vi "Asynchronous - Update Cyclic Labels Parameters Channels.vi"(5 "Channel Data []":T5[](array[typedef])=[{"Labels Settings"=[{"Name"="", "xmlName"="", "Label"=0, "transferPeriod"=0, "SDI_Enabled"=FALSE, "SDI"=0, "Word"={"Param Setting"={"Start Bit"=[], "Num Bits"=[], "Signed?"=[], "ScaleFac"=[], "ScaleOffset"=[], "Block Data Refs"=[], "Encoding"=[], "Values Array"=[], "Item Refs"=[]}}, "TransferType"=enum."ScheduledLabel", "has timestamp?"=FALSE, "Label Disable/Trigger Channel Reference"=0, "Message Handle"=0, "Initialized?"=FALSE, "Word Initial Raw Value"=0, "Label Timestamp Channel Data Reference"=0}], "channel handle"=0, "channel #"=0}] {"Labels Settings"."Label Timestamp Channel Data Reference" format="%.0x"; "Labels Settings"."Label Disable/Trigger Channel Reference" format="%.0x"; "Labels Settings"."Word"."Param Setting"."Item Refs" format="%.0x"; "Labels Settings"."Word"."Param Setting"."Num Bits" min=1 max=32; "Labels Settings"."Word"."Param Setting"."Start Bit" min=8 max=31; "Labels Settings"."Label" format="%.0o"}, 6 "core handle":u64, 7 "Map":T4[](array[typedef]) {"Channel Data Reference" format="%.0x"}, 8 "Error (in)":errorcluster, 9 "Updated FIFO Index []":i32[](array[numeric]), 10 "Doubles []":dbl[](array[numeric]), 11 "Raw Values":T1) -> (0 "Error (out)":errorcluster)   [LabVIEW 2020]
uses:
  Shared/Controls and Global/RT HW Channel.ctl
  Shared/Controls and Global/RT Label Settings.ctl
  Shared/Controls and Global/Label.ctl
  Shared/Controls and Global/transferPeriod.ctl
  Shared/Controls and Global/RT Word Settings.ctl
  Shared/Controls and Global/RT Param Setting.ctl
  Shared/Controls and Global/Start Bit.ctl
  Shared/Controls and Global/Number of Bits.ctl
  <vilib>/NI VeriStand/Custom Device API/Block Data Reference.ctl
  <vilib>/NI VeriStand/Custom Device API/Data Reference.ctl
  <vilib>/NI VeriStand/Custom Device API/Custom Device Item Ref.ctl
  Shared/Controls and Global/TransferType.ctl
  RT Controls/RT Tx Association.ctl
  RT Controls/RT Tx Default Raw Value.ctl
  RT Controls/RT Tx Default Raw Value_Association.ctl
  Insert BCD Parameter.vi
  Ballard Arinc-429 Engine.lvlib
  <instrlib>/BTI429Lib/BTI429LV.lvlib
  <vilib>/NI VeriStand/Custom Device Tools/Custom Device Utility Library/Custom Device Utility Library.lvlib
  Shared/Ballard Arinc-429 Shared.lvlib
  <vilib>/NI VeriStand/Custom Device API/Custom Device API.lvlib
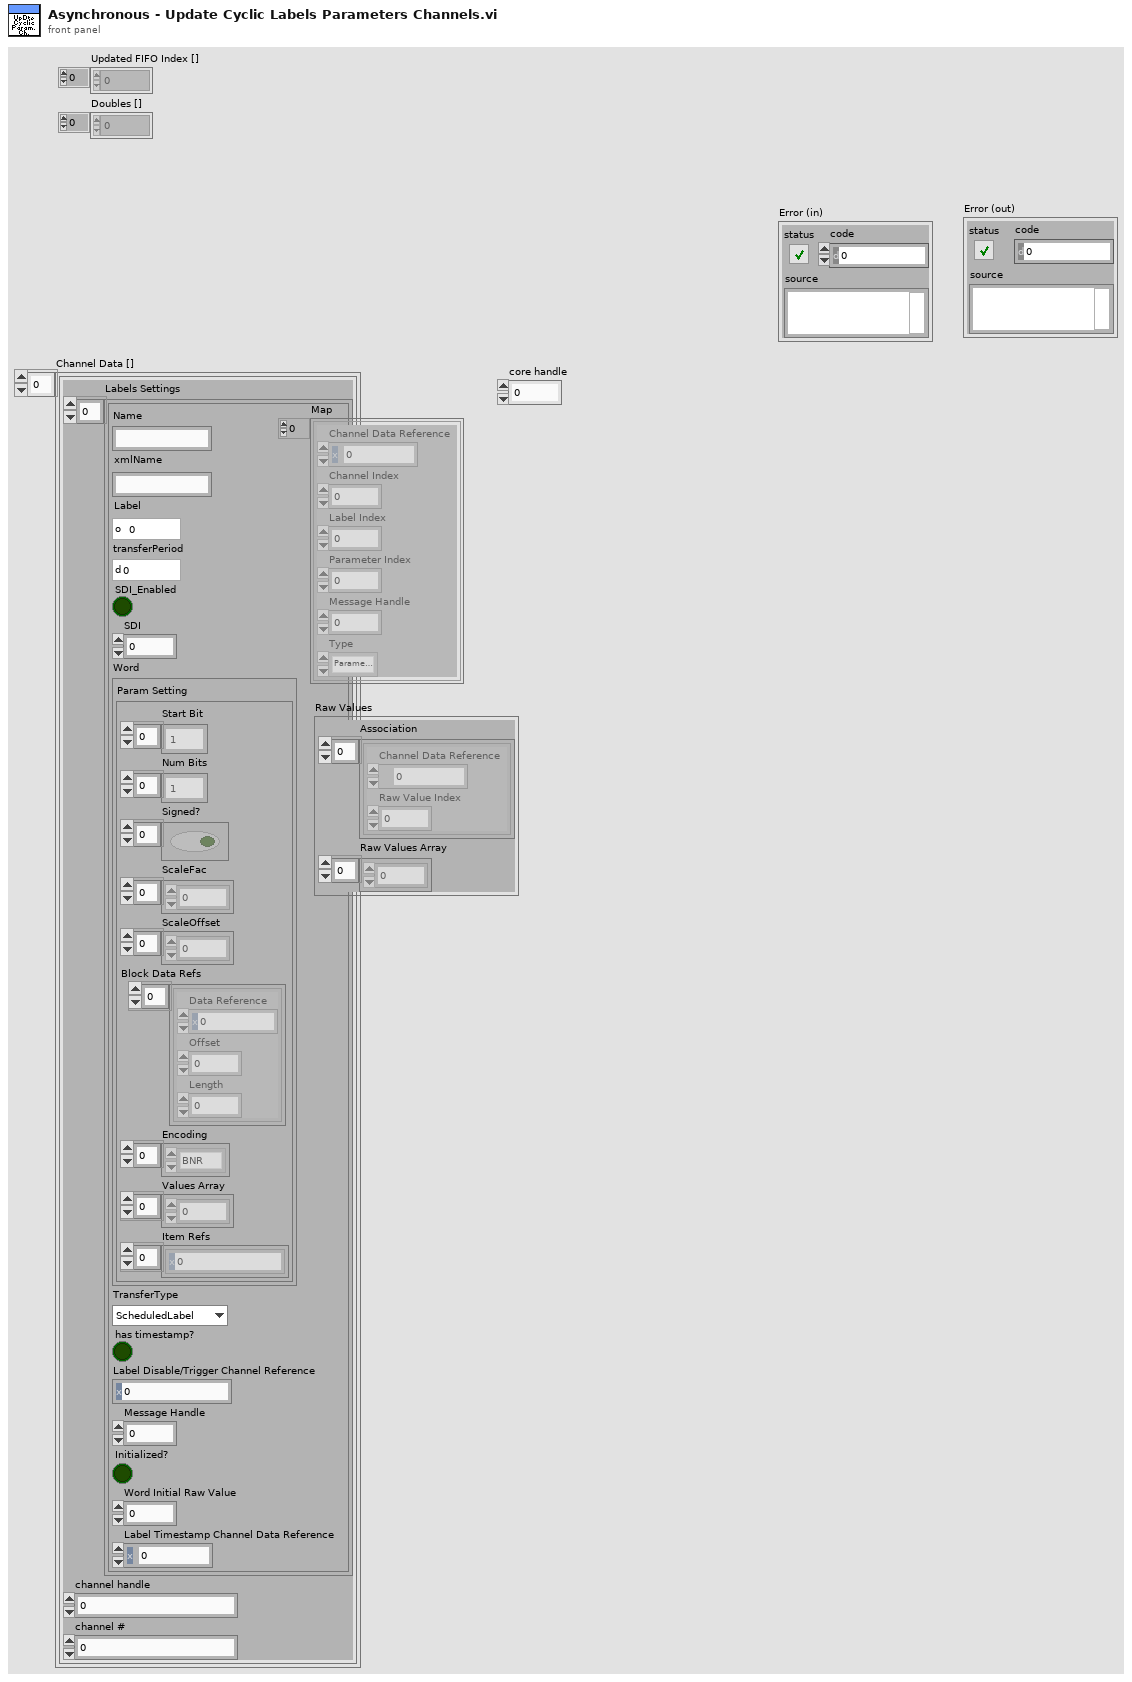
[diagram p1: front panel]
types:
  T1 = typedef "Ballard Arinc-429 Engine.lvlib/RT Tx Default Raw Value.ctl" = cluster{"Association":T2[], "Raw Values Array":u32[]}
  T2 = typedef "Ballard Arinc-429 Engine.lvlib/RT Tx Default Raw Value_Association.ctl" = cluster{"Channel Data Reference":T3, "Raw Value Index":i32}
  T3 = typedef "Custom Device API.lvlib/Data Reference.ctl" = i32
  T4 = typedef "Ballard Arinc-429 Engine.lvlib/RT Tx Association.ctl" = cluster{"Channel Data Reference":T3, "Channel Index":i32, "Label Index":i32, "Parameter Index":i32, "Message Handle":u64, "Type":enum16{"Parameter Channel", "Disable/Trigger Channel"}}
  T5 = typedef "Ballard Arinc-429 Shared.lvlib/RT HW Channel.ctl" = cluster{"Labels Settings":T6[], "channel handle":u64, "channel #":u16}
  T6 = typedef "Ballard Arinc-429 Shared.lvlib/RT Label Settings.ctl" = cluster{"Name":string, "xmlName":string, "Label":T7, "transferPeriod":T8, "SDI_Enabled":bool, "SDI":u8, "Word":T9, "TransferType":T15, "has timestamp?":bool, "Label Disable/Trigger Channel Reference":T14, "Message Handle":u64, "Initialized?":bool, "Word Initial Raw Value":u32, "Label Timestamp Channel Data Reference":T3}
  T7 = typedef "Ballard Arinc-429 Shared.lvlib/Label.ctl" = u8
  T8 = typedef "Ballard Arinc-429 Shared.lvlib/transferPeriod.ctl" = u32
  T9 = typedef "Ballard Arinc-429 Shared.lvlib/RT Word Settings.ctl" = cluster{"Param Setting":T10}
  T10 = typedef "Ballard Arinc-429 Shared.lvlib/RT Param Setting.ctl" = cluster{"Start Bit":T11[], "Num Bits":T12[], "Signed?":bool[], "ScaleFac":dbl[], "ScaleOffset":dbl[], "Block Data Refs":T13[], "Encoding":enum16{"BNR", "BCD", "Discrete"}[], "Values Array":dbl[], "Item Refs":T14[]}
  T11 = typedef "Ballard Arinc-429 Shared.lvlib/Start Bit.ctl" = i32
  T12 = typedef "Ballard Arinc-429 Shared.lvlib/Number of Bits.ctl" = i32
  T13 = typedef "Custom Device API.lvlib/Block Data Reference.ctl" = cluster{"Data Reference":T3, "Offset":u64, "Length":u64}
  T14 = typedef "Custom Device API.lvlib/Custom Device Item Ref.ctl" = u64
  T15 = typedef "Ballard Arinc-429 Shared.lvlib/TransferType.ctl" = enum16{"ScheduledLabel", "Acyclic", "Block", "Strobe"}
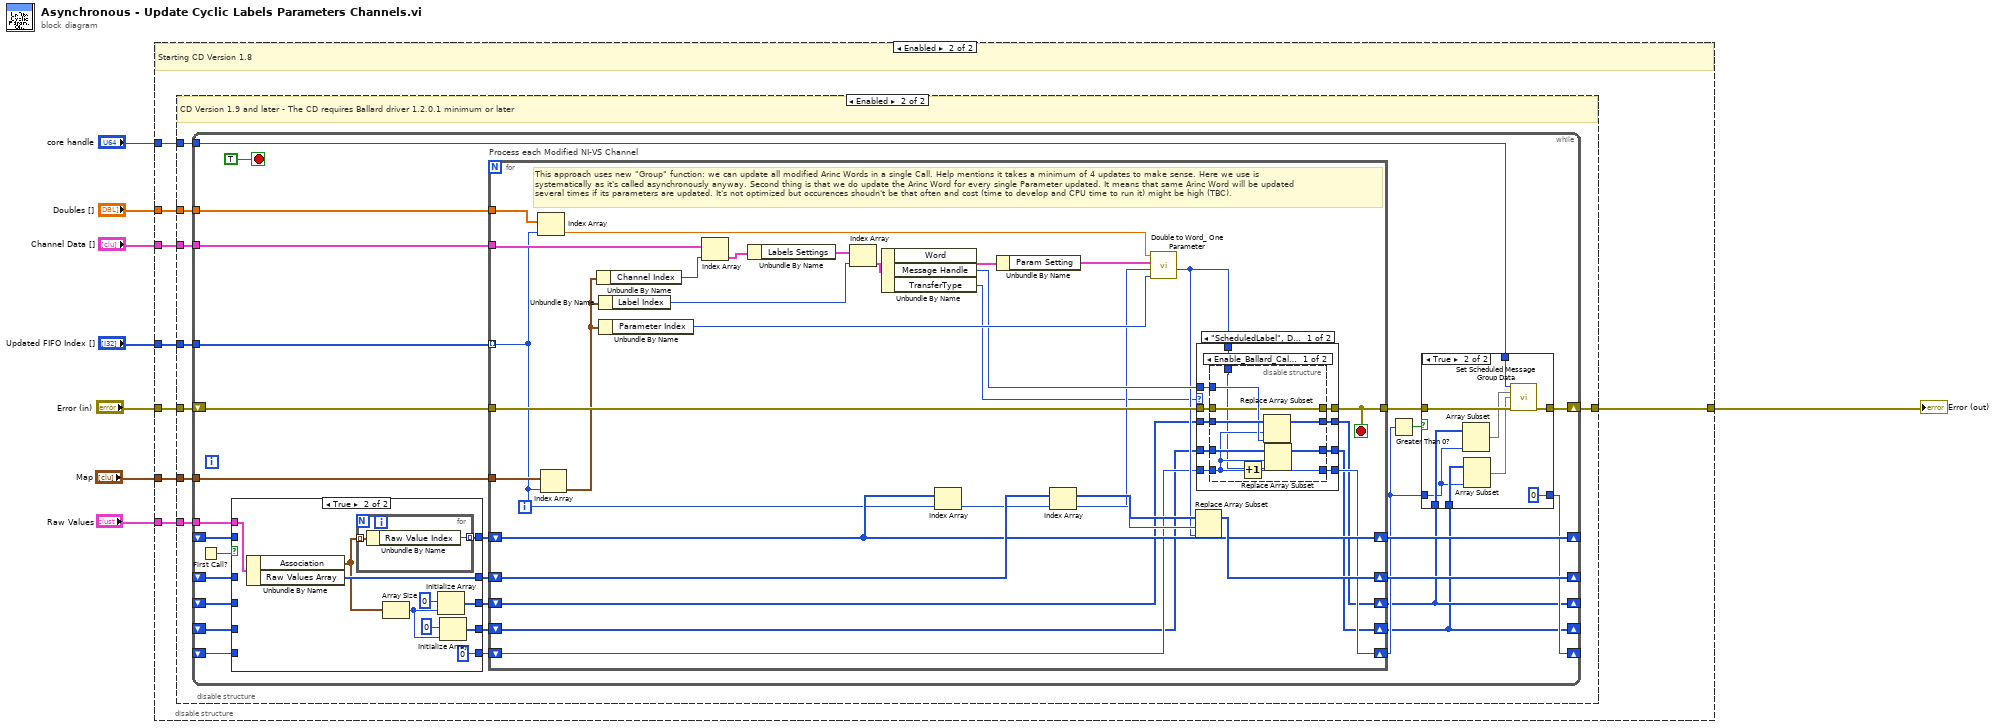
[diagram p0: block diagram]
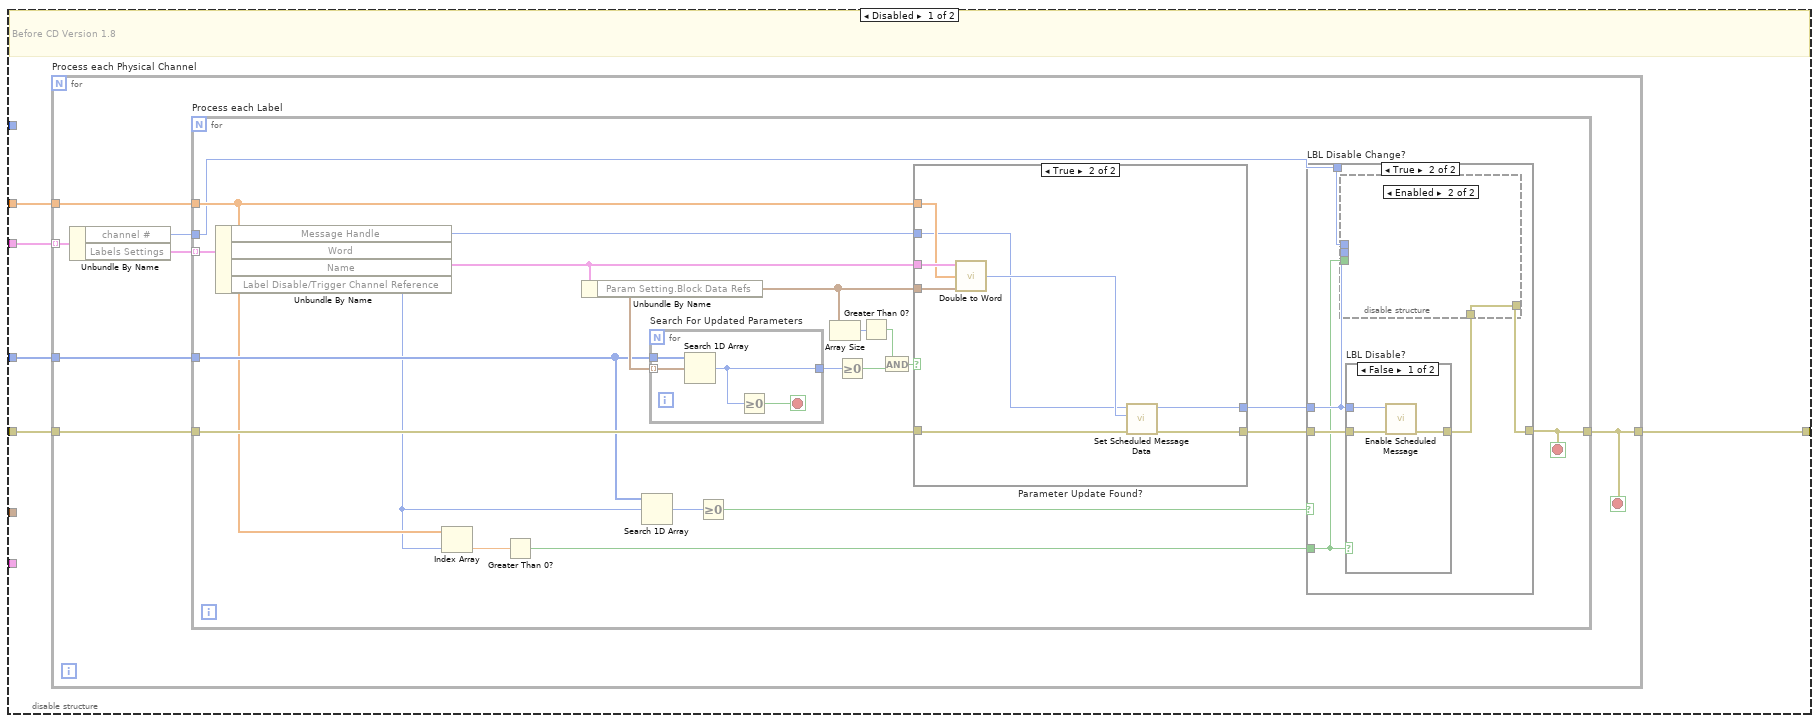
[diagram p2: hidden frame]
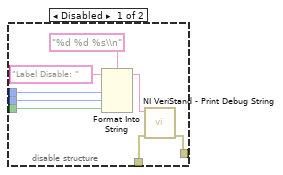
[diagram p4: hidden frame]
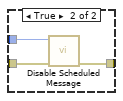
[diagram p5: hidden frame]
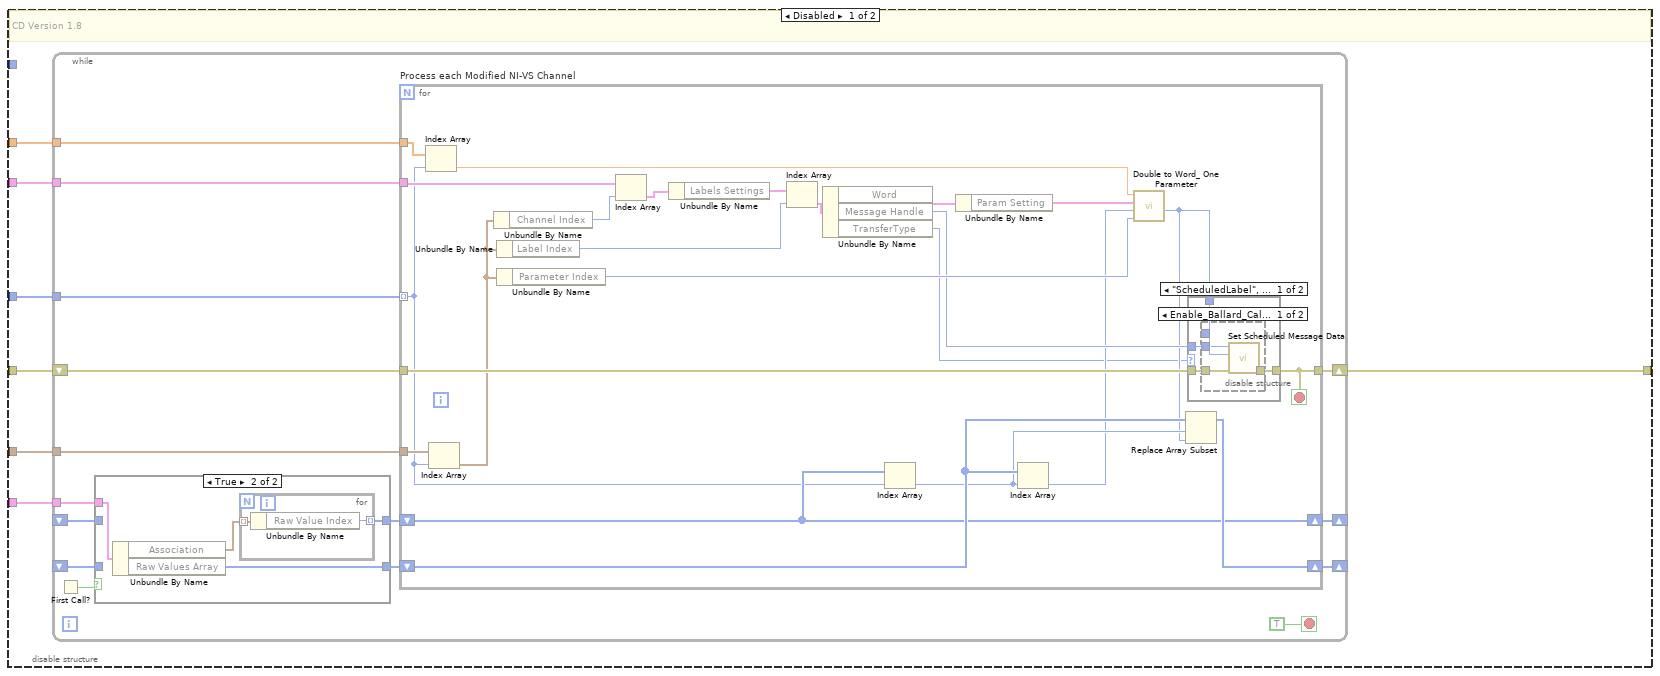
[diagram p7: hidden frame]
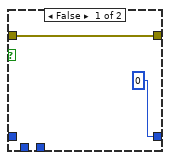
[diagram p11: hidden frame]
diagram:
  n1 = disable-structure shown="Enabled" {
    disable-tunnel: "Channel Data []" -> [w13 w85]
    disable-tunnel: "Updated FIFO Index []" -> [w12 w84]
    disable-tunnel: "Error (in)" -> [w11 w83]
    disable-tunnel: [w10 w82] -> w5
    disable-tunnel: "Doubles []" -> [w9 w81]
    disable-tunnel: "Map" -> [_ w80]
    disable-tunnel: "Raw Values" -> [_ w79]
    disable-tunnel: "core handle" -> [_ w78]
    frame Disabled {
      # "Before CD Version 1.8"
      n2 = for "Process each Physical Channel" {
        tunnel: w13 -> [w20] mode=indexing
        tunnel: w12 -> [w18]
        tunnel: w9 -> [w17]
        tunnel: w11 -> [w16]
        tunnel: [w15] -> w10
        stop <- w15 stop-if-true
        n3 = Unbundle By Name(w20) -> ("channel #"=w14:u16, "Labels Settings"=w19:T6[])
        n4 = for "Process each Label" {
          tunnel: w19 -> [w41] mode=indexing
          tunnel: w18 -> [w33]
          tunnel: w17 -> [w28]
          tunnel: [w30] -> w15
          tunnel: w16 -> [w39]
          tunnel: w14 -> [w22]
          stop <- w30 stop-if-true
          n5 = Unbundle By Name(w41) -> ("Message Handle"=w23:u64, "Word"=w21:T9, "Label Disable/Trigger Channel Reference"=w27:T14)  [unwired: 1 out]
          n6 = Index Array(array=w28, index=w27) -> (element=w26:dbl)
          n7 = Greater Than 0?(x=w26) -> (x > 0?=w25:bool)
          n8 = Unbundle By Name(w21) -> ("Param Setting.Block Data Refs"=w38:T13[])
          n9 = Search 1D Array(1D array=w33, element=w27) -> (index of element=w32:i32)  [unwired: 1 in]
          n10 = for "Search For Updated Parameters" {
            tunnel: w33 -> [w77]
            tunnel: w38 -> [w76] mode=indexing
            tunnel: [w75] -> w40
            stop <- w74 stop-if-true
            n11 = Search 1D Array(1D array=w77, element=w76) -> (index of element=w75:i32)  [unwired: 1 in]
            n12 = Greater Or Equal To 0?(x=w75) -> (x >= 0?=w74:bool)
          }
          n13 = Greater Or Equal To 0?(x=w32) -> (x >= 0?=w31:bool)
          n14 = Array Size(array=w38) -> (size(s)=w37:i32)
          n15 = Greater Or Equal To 0?(x=w40) -> (x >= 0?=w35:bool)
          n16 = Greater Than 0?(x=w37) -> (x > 0?=w36:bool)
          n17 = And(x=w36, y=w35) -> (x .and. y?=w34:bool)
          n18 = case "Parameter Update Found?" shown="True" w34 {
            tunnel: w28 -> [_ w69]
            tunnel: w21 -> [_ w73]
            tunnel: w39 -> [w65 w68]
            tunnel: [w65 w72] -> w29
            tunnel: w38 -> [_ w70]
            tunnel: w23 -> [w64 w67]
            tunnel: [w64 w66] -> w24
            frame False {
            }
            frame True {
              n19 = call "Double to Word.vi"("Word"=w73, "Doubles In []"=w69, "Channel FIFO Buffer Index"=w70) -> ("Word"=w71:u32)  [unwired: 12 in]
              n20 = call <instrlib>:"Set Scheduled Message Data.vi"("error in (no error)"=w68, "value"=w71, "message handle in"=w67) -> ("error out"=w72:errorcluster, "message handle out"=w66:u64)  [unwired: 7 in]
            }
          }
          n21 = case "LBL Disable Change?" shown="True" w31 {
            tunnel: [w42 w47] -> w30
            tunnel: w29 -> [w42 w48]
            tunnel: w25 -> [_ w43]
            tunnel: w24 -> [_ w44]
            tunnel: w22 -> [_ w45]
            frame False {
            }
            frame True {
              n22 = case "LBL Disable?" shown="False" w43 {
                tunnel: [w60 w63] -> w46
                tunnel: w48 -> [w59 w62]
                tunnel: w44 -> [w58 w61]
                frame False {
                  n23 = call <instrlib>:"Enable Scheduled Message.vi"("error in (no error)"=w59, "message handle in"=w58) -> ("error out"=w60:errorcluster)  [unwired: 8 in, 1 out]
                }
                frame True {
                  n24 = call <instrlib>:"Disable Scheduled Message.vi"("error in (no error)"=w62, "message handle in"=w61) -> ("error out"=w63:errorcluster)  [unwired: 8 in, 1 out]
                }
              }
              n25 = disable-structure shown="Enabled" {
                disable-tunnel: [w56 w57] -> w47
                disable-tunnel: w46 -> [w55 w57]
                disable-tunnel: w45 -> [w52 _]
                disable-tunnel: w44 -> [w51 _]
                disable-tunnel: w43 -> [w50 _]
                frame Disabled {
                  n26 = Format Into String(format string="%d %d %s\\n", initial string="Label Disable: ", w52, w51, w50) -> (resulting string=w53:string)  [unwired: 1 in, 1 out]
                  n27 = call <vilib>:"NI VeriStand - Print Debug String.vi"("error in (no error)"=w55, "Message"=w53) -> ("error out"=w56:errorcluster)  [unwired: 9 in]
                }
                frame Enabled {
                }
              }
            }
          }
        }
      }
    }
    frame Enabled {
      # "Starting CD Version 1.8"
      n28 = disable-structure shown="Enabled" {
        disable-tunnel: w85 -> [w92 w157]
        disable-tunnel: w84 -> [w91 w156]
        disable-tunnel: w83 -> [w90 w155]
        disable-tunnel: [w89 w154] -> w82
        disable-tunnel: w81 -> [w88 w153]
        disable-tunnel: w80 -> [w87 w152]
        disable-tunnel: w79 -> [w86 w151]
        disable-tunnel: w78 -> [_ w150]
        frame Disabled {
          # "CD Version 1.8"
          n29 = while {
            tunnel: w92 -> [w107]
            tunnel: w91 -> [w106]
            tunnel: w88 -> [w103]
            tunnel: w87 -> [w102]
            shift-right: [w104] -> w89
            shift-left: w90 -> [w105]
            tunnel: w86 -> [w100]
            shift-right: [w98] -> _
            shift-left: _ -> [w97]
            shift-right: [w95] -> _
            shift-left: _ -> [w94]
            stop <- TRUE stop-if-true
            n30 = First Call?() -> (First Call?: T/F=w93:bool)
            n31 = case shown="True" w93 {
              tunnel: w100 -> [_ w113]
              tunnel: [w109 w112] -> w99
              tunnel: w97 -> [w109 _]
              tunnel: [w108 w110] -> w96
              tunnel: w94 -> [w108 _]
              frame False {
              }
              frame True {
                n32 = Unbundle By Name(w113) -> ("Association"=w111:T2[], "Raw Values Array"=w112:u32[])
                n33 = for {
                  tunnel: w111 -> [w115] mode=indexing
                  tunnel: [w114] -> w110 mode=indexing
                  n34 = Unbundle By Name(w115) -> ("Raw Value Index"=w114:i32)
                }
              }
            }
            n35 = for "Process each Modified NI-VS Channel" {
              tunnel: w107 -> [w138]
              tunnel: w106 -> [w123] mode=indexing
              tunnel: w103 -> [w128]
              tunnel: w105 -> [w139]
              tunnel: [w129] -> w104
              tunnel: w102 -> [w131]
              shift-right: [w125] -> w98
              shift-left: w99 -> [w126]
              shift-right: [w124] -> w95
              shift-left: w96 -> [w124]
              stop <- w129 stop-if-true
              n36 = Index Array(array=w128, index=w123) -> (element=w127:dbl)
              n37 = Index Array(array=w131, index=w123) -> (element=w117:T4)
              n38 = Unbundle By Name(w117) -> ("Channel Index"=w137:i32)
              n39 = Unbundle By Name(w117) -> ("Label Index"=w134:i32)
              n40 = Unbundle By Name(w117) -> ("Parameter Index"=w132:i32)
              n41 = Index Array(array=w138, index=w137) -> (element=w136:T5)
              n42 = Unbundle By Name(w136) -> ("Labels Settings"=w135:T6[])
              n43 = Index Array(array=w135, index=w134) -> (element=w133:T6)
              n44 = Unbundle By Name(w133) -> ("Word"=w130:T9, "Message Handle"=w121:u64, "TransferType"=w116:T15)
              n45 = Index Array(array=w124, index=w123) -> (element=w122:i32)
              n46 = Unbundle By Name(w130) -> ("Param Setting"=w119:T10)
              n47 = Index Array(array=w126, index=w122) -> (element=w118:u32)
              n48 = call "Double to Word_ One Parameter.vi"("Parameter Index"=w132, "Word In"=w118, "Param Setting"=w119, "NI-VS Channel"=w127) -> ("Word Out"=w120:u32)  [unwired: 5 in]
              n49 = Replace Array Subset(array=w126, new element=w120, index=w122) -> (w125:u32[])
              n50 = case shown="\"ScheduledLabel\", Default" w116 {
                tunnel: w139 -> [w143 w149]
                tunnel: [w142 w149] -> w129
                tunnel: w121 -> [w141 _]
                tunnel: w120 -> [w140 _]
                frame "ScheduledLabel", Default {
                  n51 = disable-structure shown="Enable_Ballard_Calls==True, Default" {
                    disable-tunnel: w143 -> [w147 w148]
                    disable-tunnel: [w146 w148] -> w142
                    disable-tunnel: w140 -> [w145 _]
                    disable-tunnel: w141 -> [w144 _]
                    frame condition #0 (active) {
                      n52 = call <instrlib>:"Set Scheduled Message Data.vi"("error in (no error)"=w147, "value"=w145, "message handle in"=w144) -> ("error out"=w146:errorcluster)  [unwired: 7 in, 1 out]
                    }
                    frame condition #1 {
                    }
                  }
                }
                frame "Acyclic" {
                }
              }
            }
          }
        }
        frame Enabled {
          # "CD Version 1.9 and later - The CD requires Ballard driver 1.2.0.1 minimum or later"
          n53 = while {
            tunnel: w157 -> [w185]
            tunnel: w156 -> [w184]
            tunnel: w153 -> [w182]
            tunnel: w152 -> [w181]
            shift-right: [w164] -> w154
            shift-left: w155 -> [w183]
            tunnel: w151 -> [w179]
            shift-right: [w177] -> _
            shift-left: _ -> [w176]
            shift-right: [w174] -> _
            shift-left: _ -> [w173]
            shift-right: [w160] -> _
            shift-left: _ -> [w170]
            shift-right: [w159] -> _
            shift-left: _ -> [w168]
            shift-right: [w161] -> _
            shift-left: _ -> [w166]
            tunnel: w150 -> [w158]
            stop <- TRUE stop-if-true
            n54 = First Call?() -> (First Call?: T/F=w172:bool)
            n55 = case shown="True" w172 {
              tunnel: w179 -> [_ w211]
              tunnel: [w201 w210] -> w178
              tunnel: w176 -> [w201 _]
              tunnel: [w200 w209] -> w175
              tunnel: w173 -> [w200 _]
              tunnel: [w199 w206] -> w171
              tunnel: w170 -> [w199 _]
              tunnel: [w198 w205] -> w169
              tunnel: w168 -> [w198 _]
              tunnel: [w197 0] -> w167
              tunnel: w166 -> [w197 _]
              frame False {
              }
              frame True {
                n56 = Unbundle By Name(w211) -> ("Association"=w203:T2[], "Raw Values Array"=w210:u32[])
                n57 = for {
                  tunnel: w203 -> [w213] mode=indexing
                  tunnel: [w212] -> w209 mode=indexing
                  n58 = Unbundle By Name(w213) -> ("Raw Value Index"=w212:i32)
                }
                n59 = Array Size(array=w203) -> (size(s)=w202:i32)
                n60 = Initialize Array(u64 0, w202) -> (w206:u64[])
                n61 = Initialize Array(u32 0, w202) -> (w205:u32[])
              }
            }
            n62 = for "Process each Modified NI-VS Channel" {
              tunnel: w185 -> [w242]
              tunnel: w184 -> [w227] mode=indexing
              tunnel: w182 -> [w232]
              tunnel: w183 -> [w243]
              tunnel: [w233] -> w165
              tunnel: w181 -> [w235]
              shift-right: [w229] -> w177
              shift-left: w178 -> [w230]
              shift-right: [w228] -> w174
              shift-left: w175 -> [w228]
              shift-right: [w215] -> w160
              shift-left: w171 -> [w217]
              shift-right: [w214] -> w159
              shift-left: w169 -> [w216]
              shift-right: [w218] -> w162
              shift-left: w167 -> [w219]
              stop <- w233 stop-if-true
              # "This approach uses new \"Group\" function: we can update all modified Arinc Words in a single Call. Help mentions it takes a minimum of 4 updates to make sense. Here we use is\nsystematically as it's called asynchronously anyway. Second thing is that we do update the Arinc Word for every single Parameter updated. It means that same Arinc Word will be updated\nseveral times if its parameters are updated. It's not optimized but occurences shoudn't be that often and cost (time to develop and CPU time to run it) might be high (TBC)."
              n63 = Index Array(array=w232, index=w227) -> (element=w231:dbl)
              n64 = Index Array(array=w235, index=w227) -> (element=w221:T4)
              n65 = Unbundle By Name(w221) -> ("Channel Index"=w241:i32)
              n66 = Unbundle By Name(w221) -> ("Label Index"=w238:i32)
              n67 = Unbundle By Name(w221) -> ("Parameter Index"=w236:i32)
              n68 = Index Array(array=w242, index=w241) -> (element=w240:T5)
              n69 = Unbundle By Name(w240) -> ("Labels Settings"=w239:T6[])
              n70 = Index Array(array=w239, index=w238) -> (element=w237:T6)
              n71 = Unbundle By Name(w237) -> ("Word"=w234:T9, "Message Handle"=w225:u64, "TransferType"=w220:T15)
              n72 = Index Array(array=w228, index=w227) -> (element=w226:i32)
              n73 = Unbundle By Name(w234) -> ("Param Setting"=w223:T10)
              n74 = Index Array(array=w230, index=w226) -> (element=w222:u32)
              n75 = call "Double to Word_ One Parameter.vi"("Parameter Index"=w236, "Word In"=w222, "Param Setting"=w223, "NI-VS Channel"=w231) -> ("Word Out"=w224:u32)  [unwired: 5 in]
              n76 = Replace Array Subset(array=w230, new element=w224, index=w226) -> (w229:u32[])
              n77 = case shown="\"ScheduledLabel\", Default" w220 {
                tunnel: w243 -> [w253 w270]
                tunnel: [w252 w270] -> w233
                tunnel: w225 -> [w251 _]
                tunnel: w224 -> [w250 _]
                tunnel: w219 -> [w249 w269]
                tunnel: [w248 w269] -> w218
                tunnel: w217 -> [w247 w268]
                tunnel: [w246 w268] -> w215
                tunnel: w216 -> [w245 w267]
                tunnel: [w244 w267] -> w214
                frame "ScheduledLabel", Default {
                  n78 = disable-structure shown="Enable_Ballard_Calls==True, Default" {
                    disable-tunnel: w253 -> [w258 w266]
                    disable-tunnel: [w258 w266] -> w252
                    disable-tunnel: w250 -> [w254 _]
                    disable-tunnel: w251 -> [w259 _]
                    disable-tunnel: w249 -> [w255 w265]
                    disable-tunnel: [w262 w265] -> w248
                    disable-tunnel: w247 -> [w261 w264]
                    disable-tunnel: [w260 w264] -> w246
                    disable-tunnel: w245 -> [w257 w263]
                    disable-tunnel: [w256 w263] -> w244
                    frame condition #0 (active) {
                      n79 = Increment(x=w255) -> (x+1=w262:i32)
                      n80 = Replace Array Subset(array=w261, new element=w259, index=w255) -> (w260:u64[])
                      n81 = Replace Array Subset(array=w257, new element=w254, index=w255) -> (w256:u32[])
                    }
                    frame condition #1 {
                    }
                  }
                }
                frame "Acyclic" {
                }
              }
            }
            n82 = Greater Than 0?(x=w162) -> (x > 0?=w163:bool)
            n83 = case shown="True" w163 {
              tunnel: w165 -> [w186 w196]
              tunnel: [w186 w195] -> w164
              tunnel: w162 -> [_ w190]
              tunnel: [0 0] -> w161
              tunnel: w160 -> [_ w193]
              tunnel: w159 -> [_ w191]
              tunnel: w158 -> [_ w188]
              frame False {
              }
              frame True {
                n84 = Array Subset(array=w193, length=w190) -> (w192:u64[])  [unwired: 1 in]
                n85 = Array Subset(array=w191, length=w190) -> (w189:u32[])  [unwired: 1 in]
                n86 = call <instrlib>:"Set Scheduled Message Group Data.vi"("core handle in"=w188, "message handles in"=w192, "values"=w189, "error in (no error)"=w196) -> ("error out"=w195:errorcluster)  [unwired: 8 in, 3 out]
              }
            }
          }
        }
      }
    }
  }
  "Error (out)" <- w5
